vi "Frame Get o.vi"(8 "error in (no error)":errorcluster, 11 "IDE simple in":refnum<class "Main Panel.lvclass">) -> (0 "error out":errorcluster, 2 "<o> Data":T1, 3 "IDE simple out":refnum<class "Main Panel.lvclass">)   [LabVIEW 2018, in "Main Panel.lvlib" / "Main Panel.lvclass"]
uses:
  Main Panel.lvclass
  Frame Analizer/frame o data.ctl
  Main Panel.lvclass/Main Panel.ctl
  Frame Analizer/Data Parser.lvclass
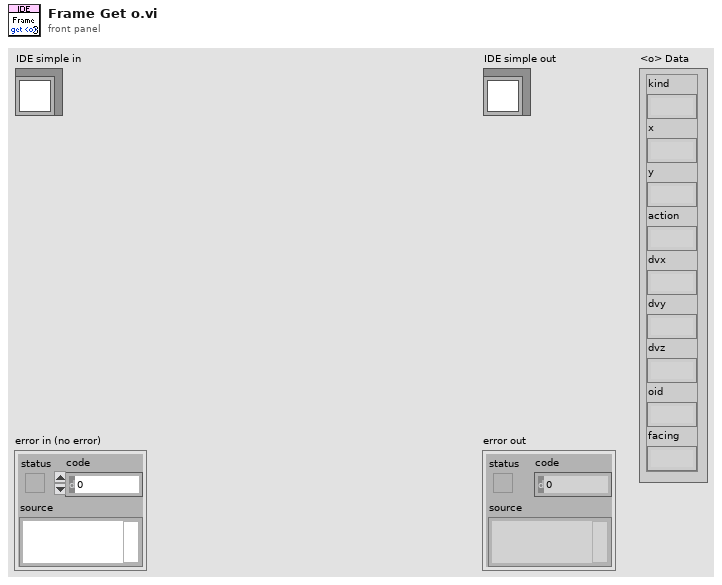
[diagram p1: front panel]
types:
  T1 = typedef "Data Parser.lvclass/frame o data.ctl" = cluster{"kind":string, "x":string, "y":string, "action":string, "dvx":string, "dvy":string, "dvz":string, "oid":string, "facing":string}
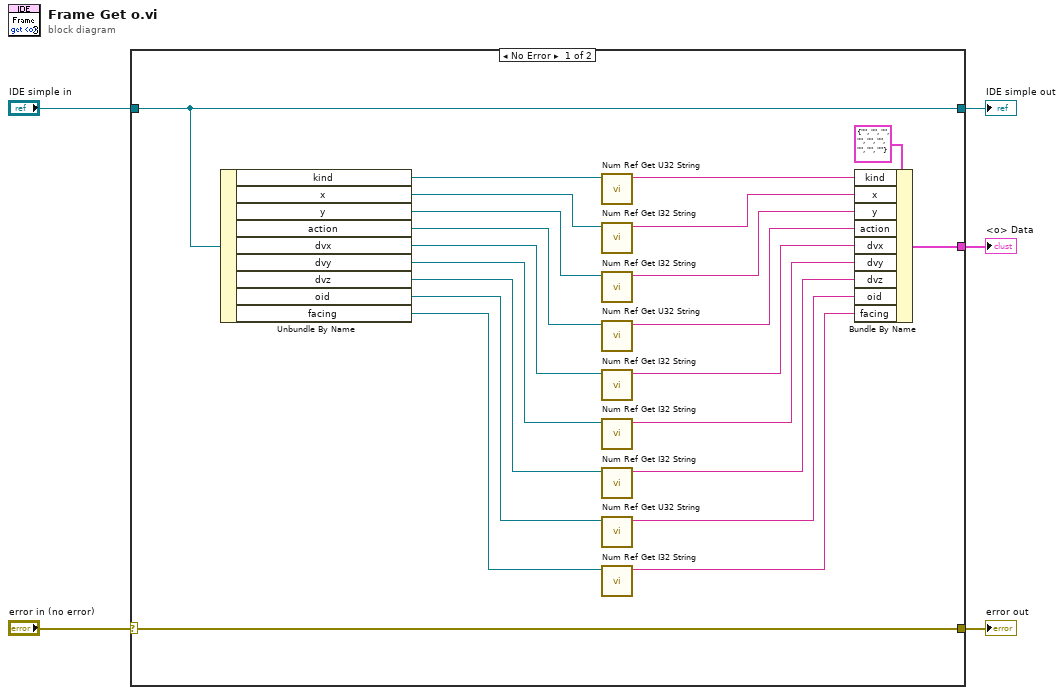
[diagram p0: block diagram]
diagram:
  n1 = case shown="No Error" "error in (no error)" {
    selector: "error in (no error)" -> [w6 w29]
    tunnel: [w6 w29] -> w4
    tunnel: [w27 w28] -> w2
    tunnel: "IDE simple in" -> [w27 w28]
    tunnel: [w26 _] -> w1
    frame No Error {
      n2 = Unbundle By Name(w27) -> ("kind"=w24:refnum<vi>, "x"=w22:refnum<vi>, "y"=w21:refnum<vi>, "action"=w20:refnum<vi>, "dvx"=w19:refnum<vi>, "dvy"=w18:refnum<vi>, "dvz"=w17:refnum<vi>, "oid"=w16:refnum<vi>, "facing"=w15:refnum<vi>)
      n3 = call "Num Ref Get U32 String.vi"("U32 Ref"=w24) -> ("Value string"=w23:string)  [unwired: 9 in, 1 out]
      n4 = call "Num Ref Get I32 String.vi"("I32 Ref"=w22) -> ("Value String"=w14:string)  [unwired: 9 in, 1 out]
      n5 = call "Num Ref Get I32 String.vi"("I32 Ref"=w21) -> ("Value String"=w13:string)  [unwired: 9 in, 1 out]
      n6 = call "Num Ref Get U32 String.vi"("U32 Ref"=w20) -> ("Value string"=w12:string)  [unwired: 9 in, 1 out]
      n7 = call "Num Ref Get I32 String.vi"("I32 Ref"=w19) -> ("Value String"=w11:string)  [unwired: 9 in, 1 out]
      n8 = call "Num Ref Get I32 String.vi"("I32 Ref"=w18) -> ("Value String"=w10:string)  [unwired: 9 in, 1 out]
      n9 = call "Num Ref Get I32 String.vi"("I32 Ref"=w17) -> ("Value String"=w9:string)  [unwired: 9 in, 1 out]
      n10 = call "Num Ref Get U32 String.vi"("U32 Ref"=w16) -> ("Value string"=w8:string)  [unwired: 9 in, 1 out]
      n11 = call "Num Ref Get I32 String.vi"("I32 Ref"=w15) -> ("Value String"=w7:string)  [unwired: 9 in, 1 out]
      n12 = Bundle By Name(cluster=T1 {"kind"="", "x"="", "y"="", "action"="", "dvx"="", "dvy"="", "dvz"="", "oid"="", "facing"=""} ("<o> data"), "kind"=w23, "x"=w14, "y"=w13, "action"=w12, "dvx"=w11, "dvy"=w10, "dvz"=w9, "oid"=w8, "facing"=w7) -> (w26:T1)
    }
    frame Error {
    }
  }
  "error out" <- w4
  "IDE simple out" <- w2
  "<o> Data" <- w1
